vi "Launch Module's.vi"(7 "Data Cluster In":T1, 8 "error in (no error)":errorcluster) -> (0 "error out":errorcluster, 5 "Data Cluster Out":T1)   [LabVIEW 2021, in "Hardware Selection.lvlib"]
uses:
  Hardware Selection.lvlib
  Module Data--cluster.ctl
  Host-Control's/RT Exec FGV Action.ctl
  Host-Control's/Module ID Action Enum.ctl
  Host-Control's/HW Name Enum.ctl
  <userlib>/_OpenG.lib/array/array.llb/Search 1D Array (Boolean)__ogtk.vi
  <userlib>/_OpenG.lib/array/array.llb/openg_array.lvlib
  RT Acquisition Engine/RT Acquisition Engine.lvlib
  Safety/Safety.lvlib
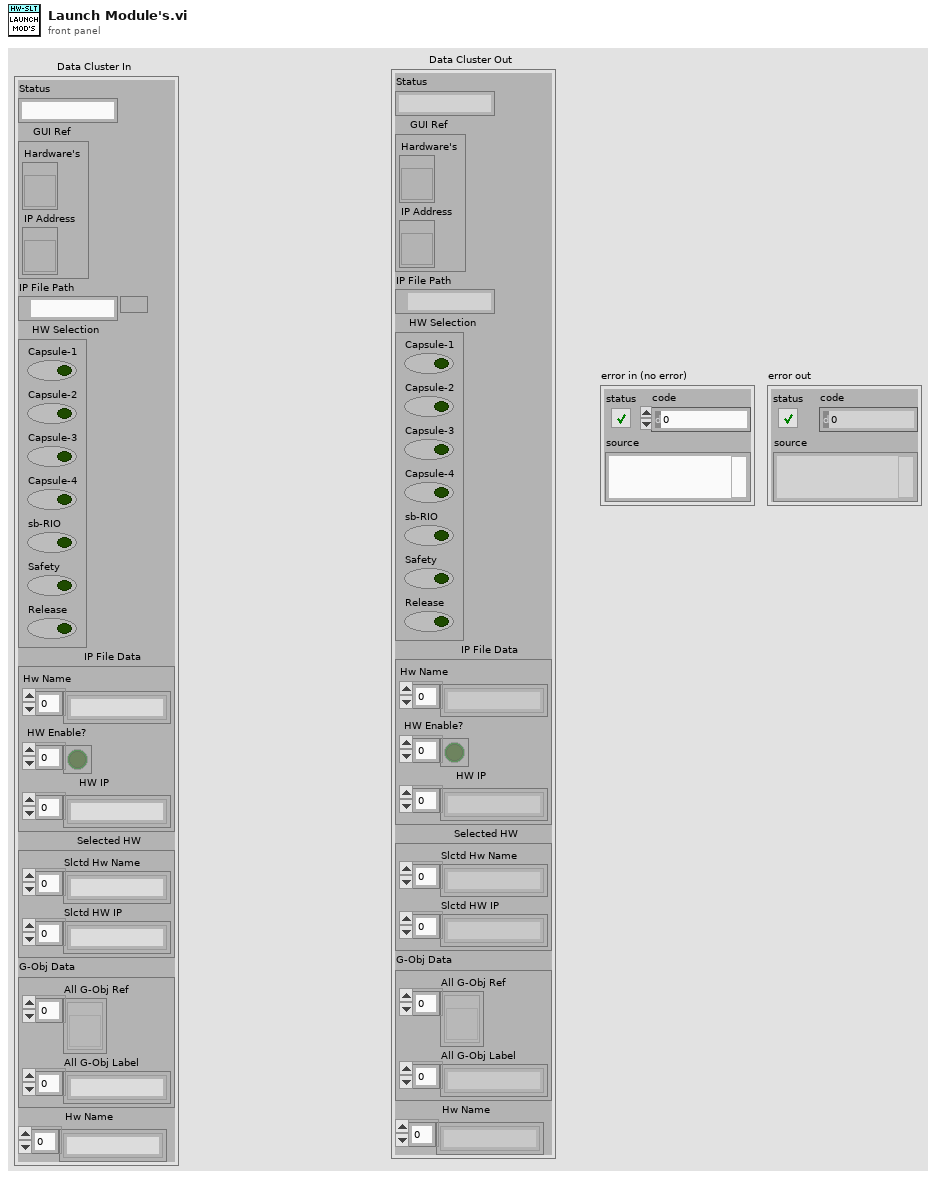
[diagram p1: front panel]
types:
  T1 = typedef "Hardware Selection.lvlib/Module Data--cluster.ctl" = cluster{"Status":string, "GUI Ref":cluster{"Hardware's":refnum<vi>, "IP Address":refnum<vi>}, "IP File Path":path, "HW Selection":cluster{"Capsule-1":bool, "Capsule-2":bool, "Capsule-3":bool, "Capsule-4":bool, "sb-RIO":bool, "Safety":bool, "Release":bool}, "IP File Data":cluster{"Hw Name":string[], "HW Enable?":bool[], "HW IP":string[]}, "Selected HW":cluster{"Slctd Hw Name":string[], "Slctd HW IP":string[]}, "G-Obj Data":cluster{"All G-Obj Ref":refnum<vi>[], "All G-Obj Label":string[]}, "Hw Name":string[]}
  T2 = cluster{"Capsule-1":bool, "Capsule-2":bool, "Capsule-3":bool, "Capsule-4":bool, "sb-RIO":bool, "Safety":bool, "Release":bool}
  T3 = typedef "Module ID Action Enum.ctl" = enum16{"Init", "Insert", "Get a ID", "Get all ID"}
  T4 = typedef "RT Exec FGV Action.ctl" = enum16{"Init", "Insert", "Get a Exec?", "Get All Exec?"}
  T5 = typedef "HW Name Enum.ctl" = enum16{"Capsule-1", "Capsule-2", "Capsule-3", "Capsule-4", "sb-RIO", "Safety", "Release"}
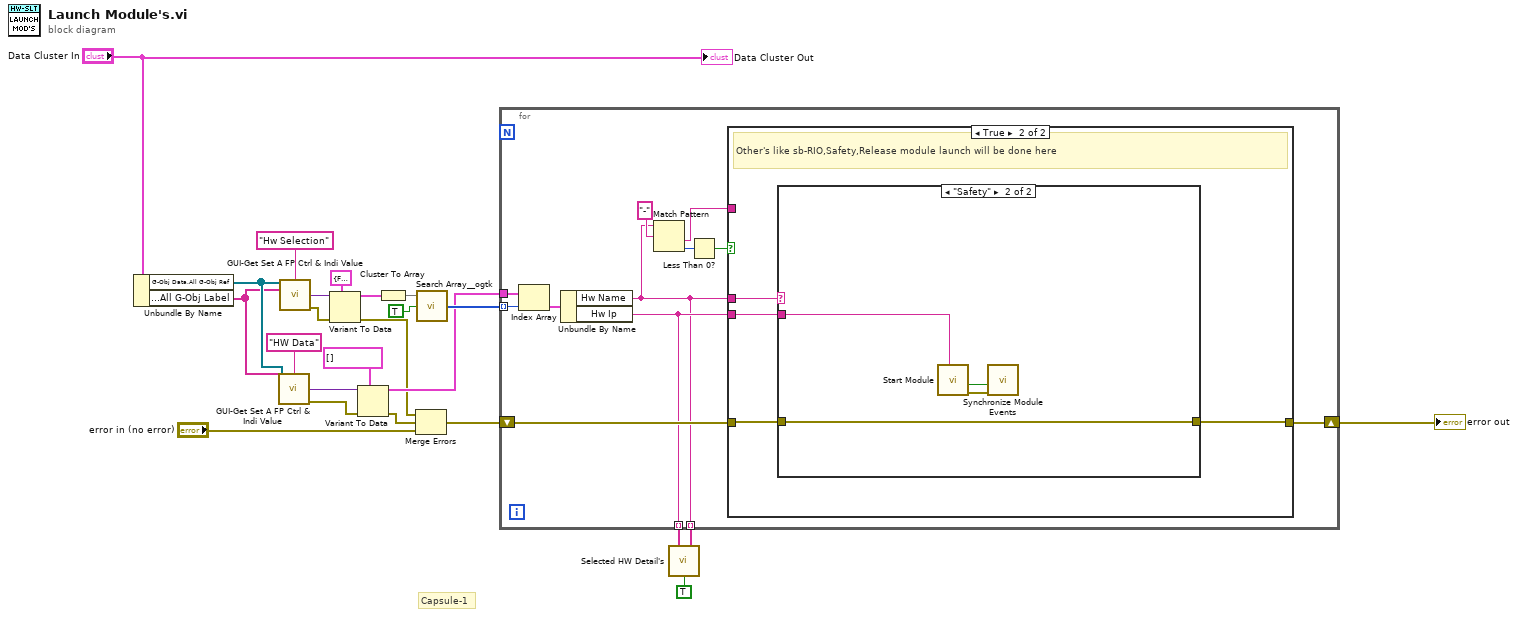
[diagram p0: block diagram]
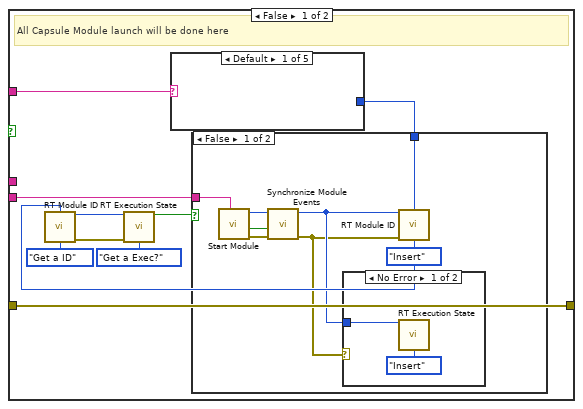
[diagram p2: hidden frame]
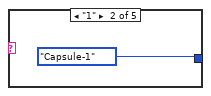
[diagram p5: hidden frame]
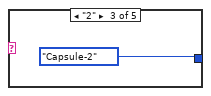
[diagram p6: hidden frame]
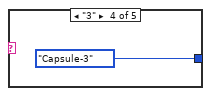
[diagram p7: hidden frame]
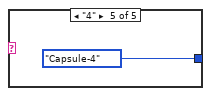
[diagram p8: hidden frame]
diagram:
  # "Capsule-1"
  n1 = Unbundle By Name("Data Cluster In") -> ("G-Obj Data.All G-Obj Ref"=w22:refnum<vi>[], "G-Obj Data.All G-Obj Label"=w21:string[])
  n2 = call "GUI-Get Set A FP Ctrl & Indi Value.vi"("All Object Ref"=w22, "Label"="HW Data", "All Object Label"=w21) -> ("Ctrl Value Out"=w20:variant, "error out"=w9:errorcluster)  [unwired: 9 in, 2 out]
  n3 = call "GUI-Get Set A FP Ctrl & Indi Value.vi"("All Object Ref"=w22, "Label"="Hw Selection", "All Object Label"=w21) -> ("Ctrl Value Out"=w19:variant, "error out"=w10:errorcluster)  [unwired: 9 in, 2 out]
  n4 = Variant To Data(error in=w10, type=T2 {"Capsule-1"=FALSE, "Capsule-2"=FALSE, "Capsule-3"=FALSE, "Capsule-4"=FALSE, "sb-RIO"=FALSE, "Safety"=FALSE, "Release"=FALSE} ("Hw Selection"), Variant=w19) -> (data=w16:T2, error out=w8:errorcluster)
  n5 = Variant To Data(error in=w9, type=cluster{"Hw Name":string, "Hw Ip":string}[] [] ("HW Data"), Variant=w20) -> (data=w12:cluster{"Hw Name":string, "Hw Ip":string}[], error out=w7:errorcluster)
  n6 = Cluster To Array(cluster=w16) -> (array=w14:bool[])
  n7 = Merge Errors(w8, w7, "error in (no error)") -> (w5:errorcluster)
  n8 = call-poly <userlib>:"Search Array__ogtk.vi"("Array"=w14, "Element Data"=TRUE) -> ("Indices of Elements"=w13:i32[])  [unwired: 7 in]
  n9 = for {
    tunnel: w13 -> [w34] mode=indexing
    tunnel: w12 -> [w35]
    shift-right: [w32] -> w4
    shift-left: w5 -> [w31]
    tunnel: [w26] -> w2 mode=indexing
    tunnel: [w25] -> w1 mode=indexing
    n10 = Index Array(array=w35, index=w34) -> (element=w33:cluster{"Hw Name":string, "Hw Ip":string})
    n11 = Unbundle By Name(w33) -> ("Hw Name"=w25:string, "Hw Ip"=w26:string)
    n12 = Match Pattern(string=w25, regular expression="-") -> (after substring=w27:string, offset past match=w29:i32)  [unwired: 1 in, 2 out]
    n13 = Less Than 0?(x=w29) -> (x < 0?=w28:bool)
    n14 = case shown="True" w28 {
      tunnel: [w44 w61] -> w32
      tunnel: w31 -> [w44 w60]
      tunnel: w25 -> [_ w62]
      tunnel: w26 -> [w43 w59]
      tunnel: w27 -> [w42 _]
      frame False {
        # "All Capsule Module launch will be done here"
        n15 = case shown="Default" w42 {
          tunnel: [_ HW_Name_Enum."Capsule-1" ("HW Name") HW_Name_Enum."Capsule-2" ("HW Name") HW_Name_Enum."Capsule-3" ("HW Name") HW_Name_Enum."Capsule-4" ("HW Name")] -> w37
          frame Default {
          }
          frame "1" {
          }
          frame "2" {
          }
          frame "3" {
          }
          frame "4" {
          }
        }
        n16 = call "RT Module ID.vi"("HW Name"=w37, "Action"=Module_ID_Action_Enum."Get a ID") -> ("Module Id Out"=w38:i32, "error out"=w39:errorcluster)  [unwired: 10 in, 2 out]
        n17 = call "RT Execution State.vi"("Module ID In"=w38, "error in"=w39, "Action"=RT_Exec_FGV_Action."Get a Exec?") -> ("Exec State? Out"=w36:bool)  [unwired: 9 in, 3 out]
        n18 = case shown="False" w36 {
          tunnel: w43 -> [w52 _]
          tunnel: w37 -> [w51 _]
          frame False {
            n19 = call "Start Module.vi"("Ip-Address"=w52) -> ("error out"=w48:errorcluster, "Wait for Event Sync?"=w49:bool, "Module ID"=w50:i32)  [unwired: 7 in, 1 out]
            n20 = call "Synchronize Module Events.vi"("error in"=w48, "Wait for Event Sync?"=w49, "Module ID in"=w50) -> ("error out"=w45:errorcluster, "Module ID out"=w46:i32)  [unwired: 7 in]
            n21 = case shown="No Error" w45 {
              tunnel: w46 -> [w53 _]
              frame No Error {
                n22 = call "RT Execution State.vi"("Module ID In"=w53, "Action"=RT_Exec_FGV_Action."Insert") -> ()  [unwired: 10 in, 4 out]
              }
              frame Error {
              }
            }
            n23 = call "RT Module ID.vi"("Module ID In"=w46, "HW Name"=w51, "error in"=w45, "Action"=Module_ID_Action_Enum."Insert") -> ()  [unwired: 8 in, 4 out]
          }
          frame True {
          }
        }
      }
      frame True {
        # "Other's like sb-RIO,Safety,Release module launch will be done here"
        n24 = case shown="\"Safety\"" w62 {
          tunnel: [w63 w67] -> w61
          tunnel: w60 -> [w63 w67]
          tunnel: w59 -> [_ w64]
          frame "False", Default {
          }
          frame "Safety" {
            n25 = call "Start Module.vi"("IP-Address"=w64) -> ("error out"=w65:errorcluster, "Wait for Event Sync?"=w66:bool)  [unwired: 7 in, 2 out]
            n26 = call "Synchronize Module Events.vi"("error in"=w65, "Wait for Event Sync?"=w66) -> ()  [unwired: 9 in, 1 out]
          }
        }
      }
    }
  }
  "error out" <- w4
  n27 = call "Selected HW Detail's.vi"("HW IP"=w2, "HW Name"=w1, "Write(F)"=TRUE) -> ()  [unwired: 10 in, 3 out]
  "Data Cluster Out" <- "Data Cluster In"
